vi "SendSqueezeRelease.vi"(0 "Queue in":refnum<queue>, 1 "threshold squeeze in":dbl, 2 "Status":refnum<vi>, 3 "ball 2":timestamp, 5 "data 1":dbl, 7 "data2":dbl, 9 "threshold release in":dbl, 12 "width squeeze in":u16, 13 "ball 1":timestamp) -> (4 "peak":bool, 6 "valley":bool, 8 "valley 2":bool, 10 "peak 2":bool, 14 "ball 1 out":timestamp, 15 "ball 2 out":timestamp)   [LabVIEW 2016]
doc: "Checks if there was a squeeze or release and sends over TCP.\ndetection is done using peak.valley point by point detection using the given width and thresholds.\nDetects only if at least 1 second passes since last detection (hardcoded in subvi)"
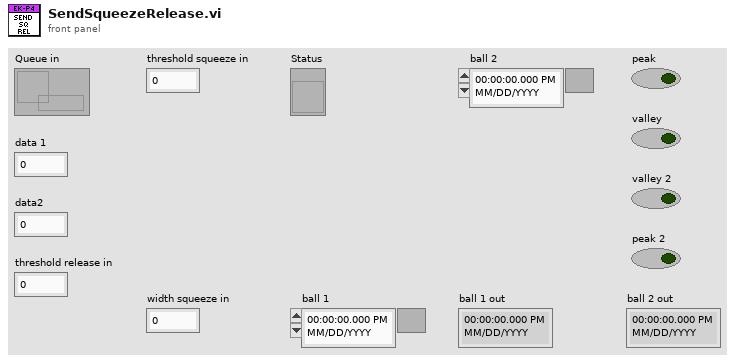
[diagram p1: front panel]
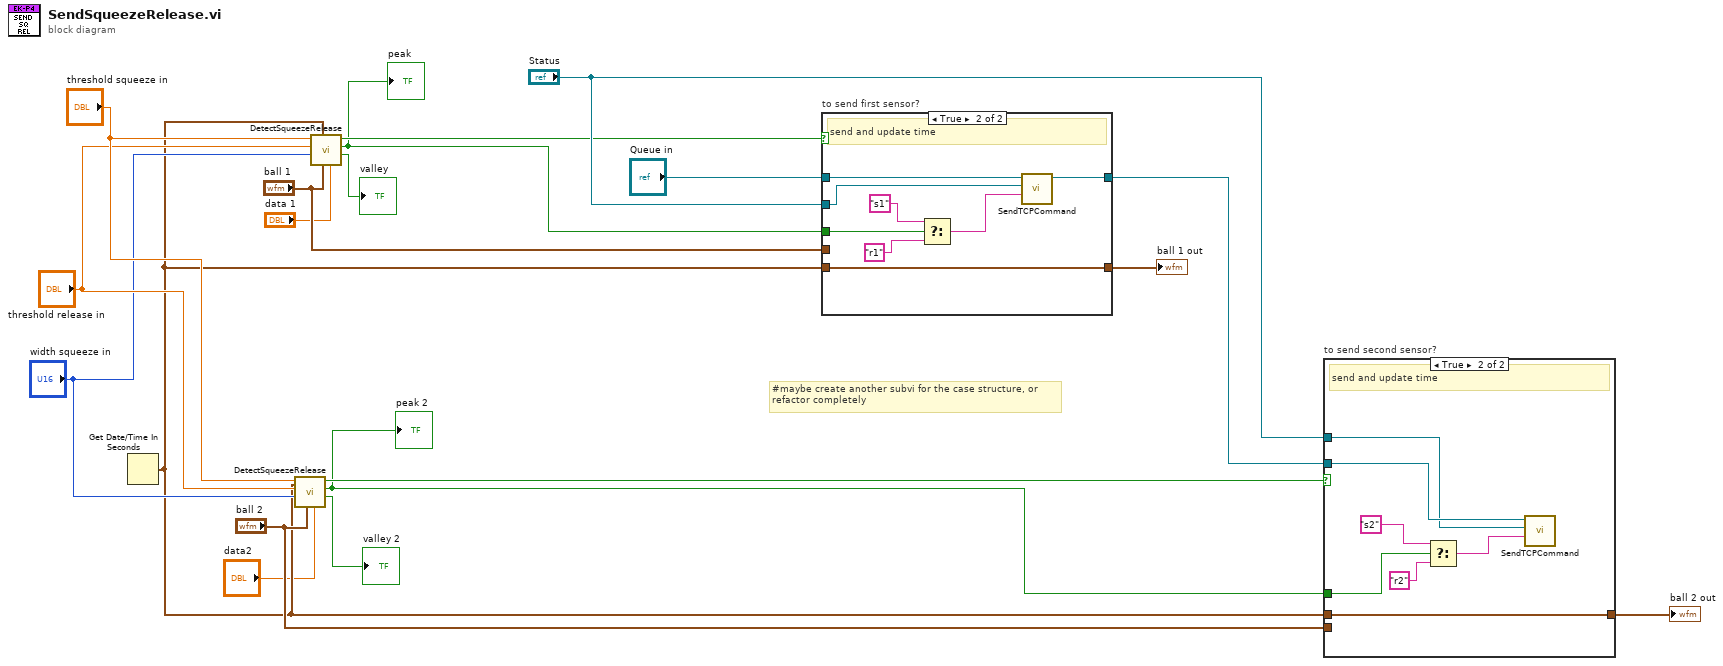
[diagram p0: block diagram]
diagram:
  # "#maybe create another subvi for the case structure, or \nrefactor completely"
  n1 = Get Date/Time In Seconds() -> (seconds since 1Jan1904=w7:timestamp)
  n2 = call "DetectSqueezeRelease.vi"("data in"="data2", "ball in"="ball 2", "Now"=w7, "width squeeze in"="width squeeze in", "threshold release in"="threshold release in", "threshold squeeze in"="threshold squeeze in") -> ("Valley out"=→"valley 2":bool, "Peak out"=w11:bool, "to send?"=w15:bool)  [unwired: 3 in]
  "peak 2" <- w11
  n3 = call "DetectSqueezeRelease.vi"("data in"="data 1", "ball in"="ball 1", "Now"=w7, "width squeeze in"="width squeeze in", "threshold release in"="threshold release in", "threshold squeeze in"="threshold squeeze in") -> ("Valley out"=→"valley":bool, "Peak out"=w2:bool, "to send?"=w4:bool)  [unwired: 3 in]
  "peak" <- w2
  n4 = case "to send first sensor?" shown="True" w4 {
    tunnel: "Queue in" -> [w21 w27]
    tunnel: "Status" -> [_ w25]
    tunnel: [w21 w24] -> w17
    tunnel: w7 -> [_ w23]
    tunnel: "ball 1" -> [w20 _]
    tunnel: [w20 w23] -> w16
    tunnel: w2 -> [_ w22]
    frame False {
      # "do nothing"
    }
    frame True {
      # "send and update time"
      n5 = Select(t="s1" ("element"), s=w22, f="r1" ("element")) -> (s? t:f=w26:string)
      n6 = call "SendTCPCommand.vi"("Command"=w26, "Status"=w25, "queue in"=w27) -> ("queue out"=w24:refnum<queue>)  [unwired: 7 in, 1 out]
    }
  }
  "ball 1 out" <- w16
  n7 = case "to send second sensor?" shown="True" w15 {
    tunnel: w11 -> [_ w37]
    tunnel: w17 -> [_ w34]
    tunnel: "Status" -> [_ w32]
    tunnel: w7 -> [_ w31]
    tunnel: [w30 w31] -> w13
    tunnel: "ball 2" -> [w30 _]
    frame False {
      # "do nothing"
    }
    frame True {
      # "send and update time"
      n8 = Select(t="s2" ("element"), s=w37, f="r2" ("element")) -> (s? t:f=w33:string)
      n9 = call "SendTCPCommand.vi"("Command"=w33, "Status"=w32, "queue in"=w34) -> ()  [unwired: 7 in, 2 out]
    }
  }
  "ball 2 out" <- w13
